vi "Read Sound ConfigurationI.vi"(8 "error constant":errorcluster, 11 "App Cfg DVR":T1) -> (0 "error out":errorcluster, 3 "Sound Manager Config":T2)   [LabVIEW 2021, in "Sound Manager.lvlib"]
doc: "This method extracts is a Poliphormic method used to read each module configuration."
uses:
  Sound Manager.lvlib
  Typedefs/Config.ctl
  Architecture/Modules/Configuration/Typedefs/App Cfg DVR.ctl
  Architecture/Typedefs/Application Configuration.ctl
  Architecture/Modules/Module Template/Typedefs/Config.ctl
  Architecture/Modules/Core UI/Typedefs/Config.ctl
  Architecture/Modules/Module Template/Module Template.lvlib
  Architecture/Modules/Core UI/Core UI.lvlib
  Architecture/Modules/Configuration/Configuration.lvlib
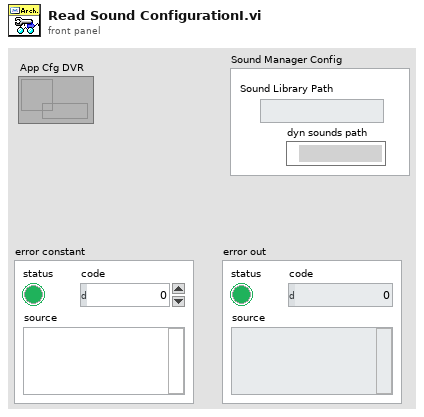
[diagram p1: front panel]
types:
  T1 = typedef "Configuration.lvlib/App Cfg DVR.ctl" = refnum<data-value>
  T2 = typedef "Sound Manager.lvlib/Config.ctl" = cluster{"Sound Library Path":path, "dyn sounds path":path}
  T3 = typedef "Configuration.lvlib/Application Configuration.ctl" = cluster{"Module Template Config":T4, "Core UI Config":T5, "Sound Manager Config":T2}
  T4 = typedef "Module Template.lvlib/Config.ctl" = cluster{"Module Enabled":bool}
  T5 = typedef "Core UI.lvlib/Config.ctl" = cluster{"Module Enabled":bool}
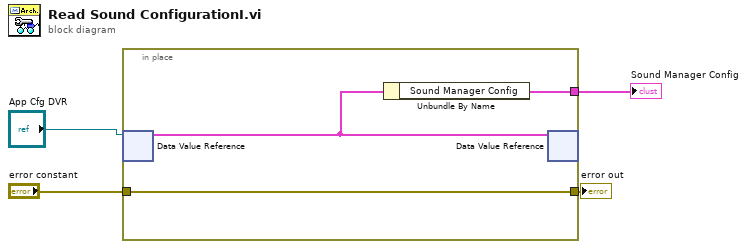
[diagram p0: block diagram]
diagram:
  n1 = in-place {
    in-place-border: "error constant" -> [w7]
    in-place-border: [w7] -> w3
    in-place-border: [w5] -> w1
    n2 = in-place-dvr #1("App Cfg DVR") -> (w6:T3)  [unwired: 1 out]
    n3 = Unbundle By Name(w6) -> ("Sound Manager Config"=w5:T2)
    n4 = in-place-dvr #1(w6) -> ()  [unwired: 2 out]
  }
  "error out" <- w3
  "Sound Manager Config" <- w1
